vi "File.Filter list by File Name Pattern.vi"(9 "AND Patterns":string[](array[string]), 10 "OR Patterns":string[](array[string]), 11 "Files":path[](array[path])) -> (3 "Filtered List":path[](array[path]))   [LabVIEW 2018]
panel:
  in  "Test Path":path
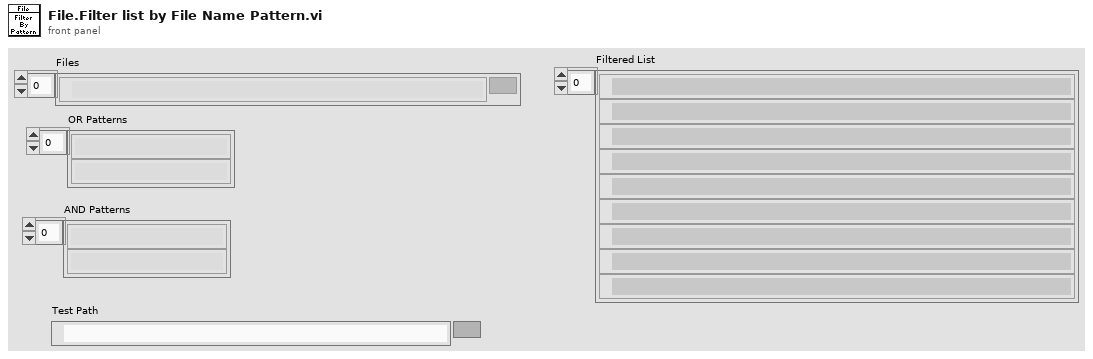
[diagram p1: front panel]
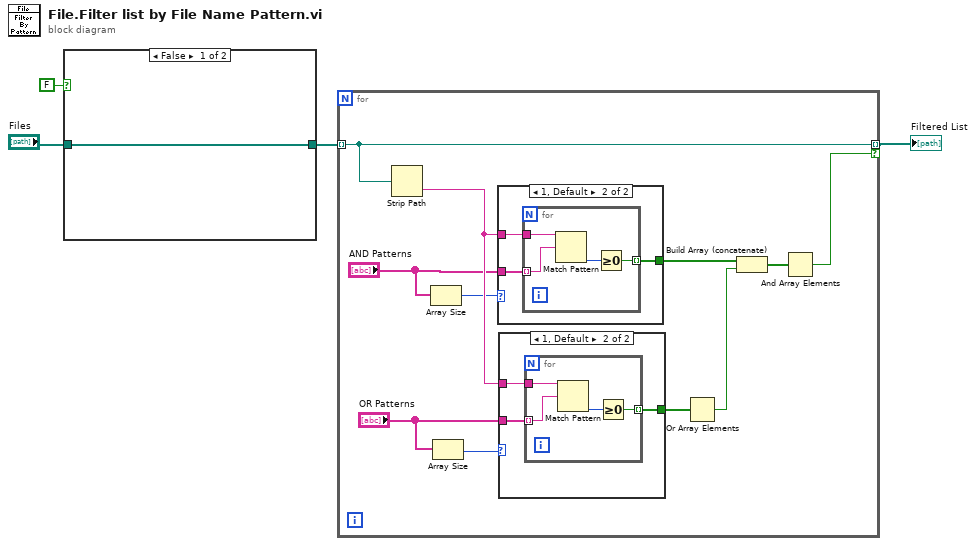
[diagram p0: block diagram]
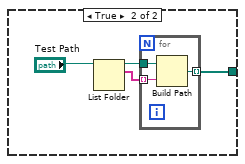
[diagram p2: hidden frame]
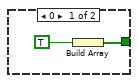
[diagram p3: hidden frame]
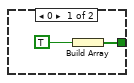
[diagram p4: hidden frame]
diagram:
  n1 = case shown="False" FALSE {
    tunnel: [w5 w6] -> w4
    tunnel: "Files" -> [w5 _]
    frame False {
    }
    frame True {
      n2 = List Folder(path="Test Path") -> (path out=w8:path, filenames=w7:string[])  [unwired: 3 in, 2 out]
      n3 = for {
        tunnel: w8 -> [w12]
        tunnel: w7 -> [w11] mode=indexing
        tunnel: [w10] -> w6 mode=indexing
        n4 = Build Path(base path=w12, name or relative path=w11) -> (appended path=w10:path)
      }
    }
  }
  n5 = for {
    tunnel: w4 -> [w23] mode=indexing
    tunnel: [w23] -> w3 mode=indexing if=w13
    n6 = Strip Path(path=w23) -> (name=w22:string)  [unwired: 1 out]
    n7 = Array Size(array="AND Patterns") -> (size(s)=w19:i32)
    n8 = Array Size(array="OR Patterns") -> (size(s)=w17:i32)
    n9 = case shown="1, Default" w19 {
      tunnel: "AND Patterns" -> [_ w37]
      tunnel: w22 -> [_ w36]
      tunnel: [w33 w35] -> w15
      frame 0 {
        n10 = Build Array(TRUE) -> (w33:bool[])
      }
      frame 1, Default {
        n11 = for {
          tunnel: w37 -> [w40] mode=indexing
          tunnel: w36 -> [w41]
          tunnel: [w38] -> w35 mode=indexing
          n12 = Match Pattern(string=w41, regular expression=w40) -> (offset past match=w39:i32)  [unwired: 1 in, 3 out]
          n13 = Greater Or Equal To 0?(x=w39) -> (x >= 0?=w38:bool)
        }
      }
    }
    n14 = case shown="1, Default" w17 {
      tunnel: w22 -> [_ w28]
      tunnel: [w24 w27] -> w21
      tunnel: "OR Patterns" -> [_ w26]
      frame 0 {
        n15 = Build Array(TRUE) -> (w24:bool[])
      }
      frame 1, Default {
        n16 = for {
          tunnel: w26 -> [w31] mode=indexing
          tunnel: w28 -> [w32]
          tunnel: [w29] -> w27 mode=indexing
          n17 = Match Pattern(string=w32, regular expression=w31) -> (offset past match=w30:i32)  [unwired: 1 in, 3 out]
          n18 = Greater Or Equal To 0?(x=w30) -> (x >= 0?=w29:bool)
        }
      }
    }
    n19 = Or Array Elements(Boolean array=w21) -> (logical OR=w14:bool)
    n20 = Build Array (concatenate)(w15, w14) -> (w16:bool[])
    n21 = And Array Elements(Boolean array=w16) -> (logical AND=w13:bool)
  }
  "Filtered List" <- w3
